vi "ActionVIOnLoad.vi"(8 "error in (no error)":errorcluster, 11 "Device Item Ref in":T1 format="%.0x") -> (0 "error out":errorcluster, 3 "Device Item Ref out":T1 format="%.0x")   [LabVIEW 2019, in "Diagnostics Addon System Explorer.lvlib"]
uses:
  Diagnostics Addon System Explorer.lvlib
  <vilib>/NI VeriStand/Custom Device API/Custom Device Item Ref.ctl
  Addon Shared/SubVIs/Constants.vi
  Addon Shared/Diagnostics Addon Shared.lvlib
  <vilib>/NI VeriStand/Custom Device API/Custom Device API.lvlib
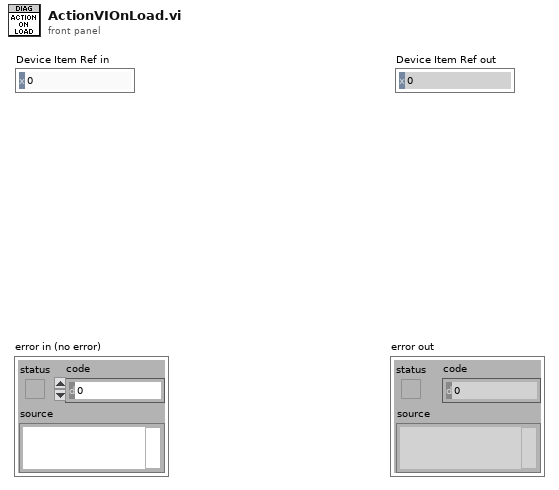
[diagram p1: front panel]
types:
  T1 = typedef "Custom Device API.lvlib/Custom Device Item Ref.ctl" = u64
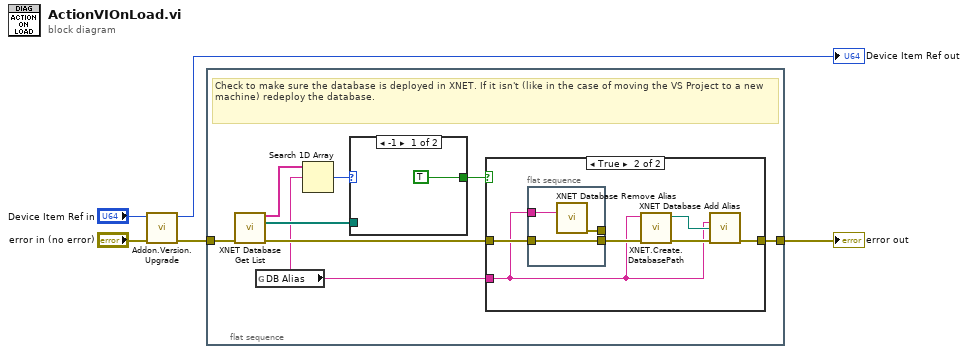
[diagram p0: block diagram]
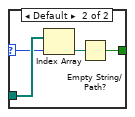
[diagram p3: hidden frame]
diagram:
  n1 = call "Addon.Version.Upgrade.vi"("error in (no error)"="error in (no error)", "Device Item Ref in in"="Device Item Ref in") -> ("error out"=w2:errorcluster, "Device Item Ref out"=→"Device Item Ref out":T1)  [unwired: 8 in]
  n2 = flat-sequence {
    tunnel: [w10] -> w3
    tunnel: w2 -> [w9]
    frame #0 {
      # "Check to make sure the database is deployed in XNET. If it isn't (like in the case of moving the VS Project to a new machine) redeploy the database."
      n3 = call <vilib>:"XNET Database Get List.vi"("error in (no error)"=w9) -> ("array of alias"=w13:string[], "array of filepath"=w12:path[], "error out"=w8:errorcluster)  [unwired: 12 in]
      n4 = global read "Constants.vi" "DB Alias"() -> (w6:string)
      n5 = Search 1D Array(1D array=w13, element=w6) -> (index of element=w11:i32)  [unwired: 1 in]
      n6 = case shown="-1" w11 {
        selector: w11 -> [_ w26]
        tunnel: w12 -> [_ w28]
        tunnel: [TRUE w25] -> w7
        frame -1 {
        }
        frame Default {
          n7 = Index Array(array=w28, index=w26) -> (element=w27:path)
          n8 = Empty String/Path?(string/path=w27) -> (empty?=w25:bool)
        }
      }
      n9 = case shown="True" w7 {
        tunnel: [w14 w16] -> w10
        tunnel: w8 -> [w14 w17]
        tunnel: w6 -> [_ w15]
        frame False {
        }
        frame True {
          n10 = flat-sequence {
            tunnel: [w23] -> w19
            tunnel: w17 -> [w23]
            tunnel: [w22] -> _
            tunnel: w15 -> [w21]
            frame #0 {
              n11 = call <vilib>:"XNET Database Remove Alias.vi"("alias"=w21) -> ("error out"=w22:errorcluster)  [unwired: 14 in]
            }
          }
          n12 = call "XNET.Create.DatabasePath.vi"("error in (no error)"=w19, "DB Alias"=w15) -> ("error out"=w20:errorcluster, "DB Path"=w18:path)  [unwired: 8 in]
          n13 = call <vilib>:"XNET Database Add Alias.vi"("alias"=w15, "filepath"=w18, "error in (no error)"=w20) -> ("error out"=w16:errorcluster)  [unwired: 12 in]
        }
      }
    }
  }
  "error out" <- w3
